vi "raw_to_calibrated_configuration-scalar.vi"(5 "tag_name":string, 7 "configuration":T1[](array[typedef]), 8 "error in (no error)":errorcluster, 11 "value in":dbl) -> (0 "error out":errorcluster, 3 "value out":dbl)   [LabVIEW 2015, in "lv-calibration.lvlib"]
uses:
  lv-calibration.lvlib
  <userlib>/antonio-alexander/lv-calibration/public/_controls/configuration.ctl
  _controls/type.ctl
  <userlib>/antonio-alexander/lv-calibration/public/_controls/point.ctl
  _controls/error.ctl
  <vilib>/gmath/NI_Gmath.lvlib
  <vilib>/Analysis/NI_AALPro.lvlib
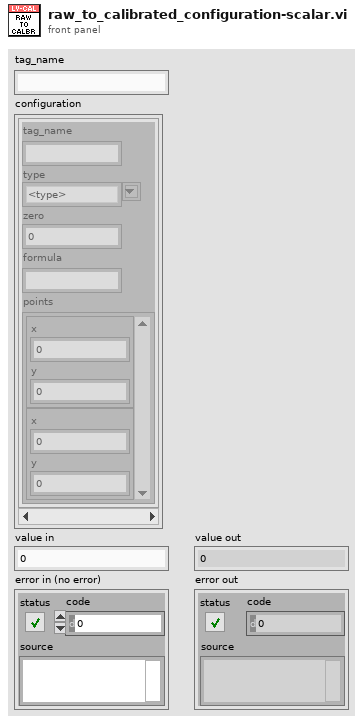
[diagram p1: front panel]
types:
  T1 = typedef "configuration.ctl" = cluster{"tag_name":string, "type":T2, "zero":dbl, "formula":string, "points":T3[]}
  T2 = typedef "lv-calibration.lvlib/type.ctl" = string
  T3 = typedef "point.ctl" = cluster{"x":dbl, "y":dbl}
  T4 = typedef "lv-calibration.lvlib/error.ctl" = enum16{"<error>", "unsupported_calibration_type", "tag_name_not_found", "duplicate_tag_names", "formula_empty"}
  T5 = typedef "lv-calibration.lvlib/runtime.ctl" = cluster{"tag_name":string, "type":T2, "offset":dbl, "slope":dbl, "formula":string, "x_points":dbl[], "y_points":dbl[]}
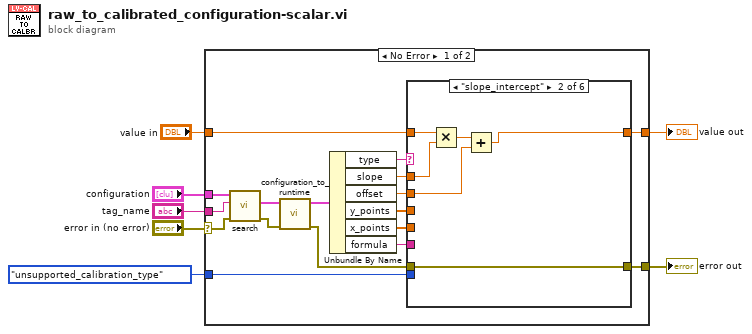
[diagram p0: block diagram]
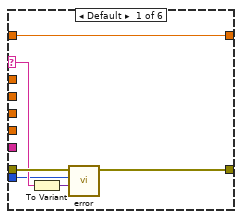
[diagram p2: hidden frame]
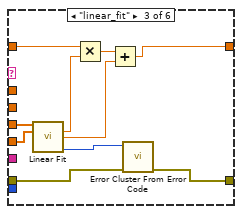
[diagram p3: hidden frame]
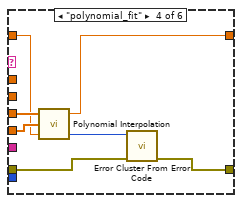
[diagram p4: hidden frame]
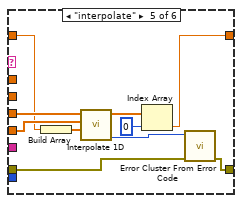
[diagram p5: hidden frame]
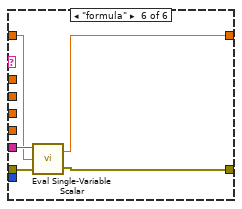
[diagram p6: hidden frame]
diagram:
  n1 = case shown="No Error" "error in (no error)" {
    selector: "error in (no error)" -> [w12 w69]
    tunnel: "value in" -> [w21 _]
    tunnel: [w20 _] -> w6
    tunnel: [w19 w69] -> w5
    tunnel: error."unsupported_calibration_type" ("error") -> [w18 _]
    tunnel: "configuration" -> [w14 _]
    tunnel: "tag_name" -> [w13 _]
    frame No Error {
      n2 = call "search.vi"("error in (no error)"=w12, "tag_name"=w13, "configuration []"=w14) -> ("error out"=w9:errorcluster, "configuration"=w11:T1)  [unwired: 6 in, 1 out]
      n3 = call "configuration_to_runtime.vi"("error in (no error)"=w9, "configuration"=w11) -> ("error out"=w8:errorcluster, "runtime"=w10:T5)  [unwired: 8 in]
      n4 = Unbundle By Name(w10) -> ("type"=w24:T2, "slope"=w23:dbl, "offset"=w22:dbl, "y_points"=w17:dbl[], "x_points"=w16:dbl[], "formula"=w15:string)
      n5 = case shown="\"slope_intercept\"" w24 {
        selector: w24 -> [w28 _ _ _ _ _]
        tunnel: w8 -> [w29 w31 w38 w48 w55 w65]
        tunnel: w23 -> [_ w35 _ _ _ _]
        tunnel: w22 -> [_ w34 _ _ _ _]
        tunnel: w21 -> [w30 w36 w42 w51 w61 w67]
        tunnel: [w30 w32 w40 w50 w58 w66] -> w20
        tunnel: [w25 w31 w37 w47 w54 w64] -> w19
        tunnel: w18 -> [w26 _ _ _ _ _]
        tunnel: w17 -> [_ _ w46 w53 w63 _]
        tunnel: w16 -> [_ _ w45 w52 w62 _]
        tunnel: w15 -> [_ _ _ _ _ w68]
        frame Default {
          n6 = To Variant(anything=w28) -> (Variant=w27:variant)
          n7 = call "error.vi"("data"=w27, "error"=w26, "error in (no error)"=w29) -> ("error out"=w25:errorcluster)  [unwired: 8 in]
        }
        frame "slope_intercept" {
          n8 = Multiply(x=w36, y=w35) -> (x*y=w33:dbl)
          n9 = Add(x=w33, y=w34) -> (x+y=w32:dbl)
        }
        frame "linear_fit" {
          n10 = call <vilib>:"Linear Fit.vi"("Y"=w46, "X"=w45) -> ("slope"=w43:dbl, "intercept"=w41:dbl, "error"=w39:i32)  [unwired: 9 in, 2 out]
          n11 = Multiply(x=w42, y=w43) -> (x*y=w44:dbl)
          n12 = Add(x=w44, y=w41) -> (x+y=w40:dbl)
          n13 = call <vilib>:"Error Cluster From Error Code.vi"("error in (no error)"=w38, "error code (0)"=w39) -> ("error out"=w37:errorcluster)  [unwired: 7 in]
        }
        frame "polynomial_fit" {
          n14 = call <vilib>:"Polynomial Interpolation.vi"("x value"=w51, "X"=w52, "Y"=w53) -> ("error"=w49:i32, "interpolation value"=w50:dbl)  [unwired: 1 out]
          n15 = call <vilib>:"Error Cluster From Error Code.vi"("error in (no error)"=w48, "error code (0)"=w49) -> ("error out"=w47:errorcluster)  [unwired: 7 in]
        }
        frame "interpolate" {
          n16 = Build Array(w61) -> (w60:dbl[])
          n17 = call <vilib>:"Interpolate 1D.vi"("xi"=w60, "X"=w62, "Y"=w63) -> ("error"=w56:i32, "yi"=w59:dbl[])  [unwired: 6 in, 1 out]
          n18 = Index Array(array=w59, index=0) -> (element=w58:dbl)
          n19 = call <vilib>:"Error Cluster From Error Code.vi"("error in (no error)"=w55, "error code (0)"=w56) -> ("error out"=w54:errorcluster)  [unwired: 7 in]
        }
        frame "formula" {
          n20 = call <vilib>:"Eval Single-Variable Scalar.vi"("error in (no error)"=w65, "x value"=w67, "formula"=w68) -> ("error out"=w64:errorcluster, "y value"=w66:dbl)
        }
      }
    }
    frame Error {
    }
  }
  "error out" <- w5
  "value out" <- w6
